vi "Variant Array to JSON Object text.vi"(5 "enable LabVIEW extensions? (T)":bool, 7 "Pretty Print?":bool, 8 "error in (no error)":errorcluster, 9 "Names":string[](array[string]), 10 "Array":variant[](array[variant])) -> (0 "error out":errorcluster, 3 "<JSON>Object Text":string)   [LabVIEW 2013, in "JSONtext.lvlib"]
uses:
  JSONtext.lvlib
  support/Tag for JSON Text.vi
  <vilib>/Utility/VariantDataType/VariantType.lvlib
  support/JSONtext support.lvlib
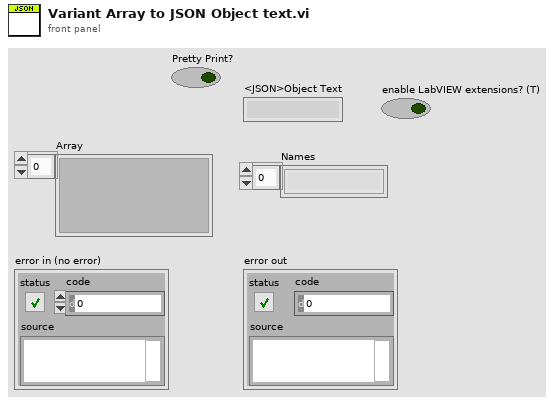
[diagram p1: front panel]
types:
  T1 = typedef "VariantType.lvlib/Type.ctl" = enum8{"Invalid Type", "Void", "I8", "I16", "I32", "I64", "U8", "U16", "U32", "U64", "Single Float", "Double Float", "Extended Float", "Single Complex", "Double Complex", "Extended Complex", "Enum U8", "Enum U16", "Enum U32", "Enum U64", "Single Float With Unit", "Double Float With Unit", "Extended Float With Unit", "Single Complex with Unit", "Double Complex with Unit", "Extended Complex with Unit", "Boolean", "String", "Path", "Picture", "Tag", "Array", "Cluster", "Variant", "LV Variant", "Waveform", "Timestamp", "Digital Waveform", "Digital Data", "ExpressData", "Refnum", "External Data", "VI", "Poly VI", "LabVIEW Class Instance", "Fixed Point"}
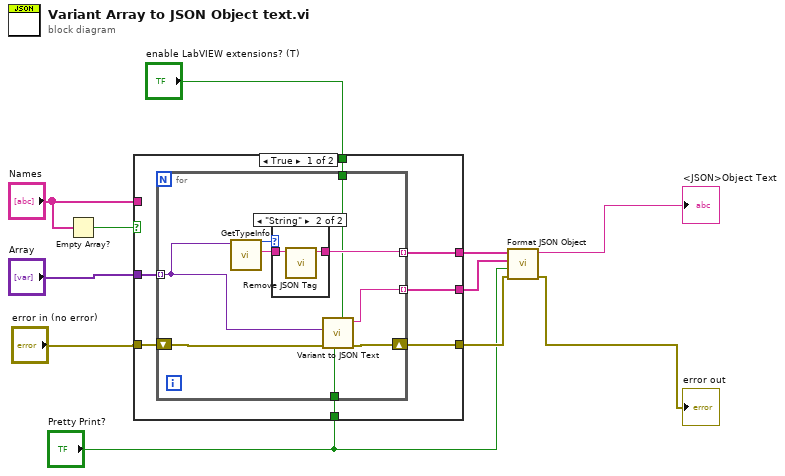
[diagram p0: block diagram]
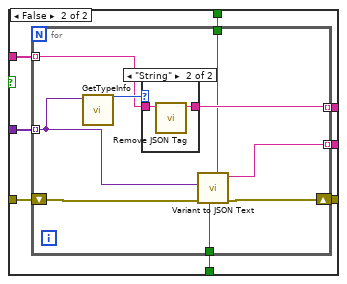
[diagram p3: hidden frame]
diagram:
  n1 = Empty Array?(array="Names") -> (empty?=w4:bool)
  n2 = case shown="True" w4 {
    tunnel: [w18 w38] -> w10
    tunnel: [w17 w37] -> w8
    tunnel: [w16 w36] -> w7
    tunnel: "error in (no error)" -> [w15 w35]
    tunnel: "Array" -> [w14 w34]
    tunnel: "Names" -> [_ w33]
    tunnel: "Pretty Print?" -> [w13 w32]
    tunnel: "enable LabVIEW extensions? (T)" -> [w12 w31]
    frame True {
      n3 = for {
        shift-right: [w23] -> w18
        shift-left: w15 -> [w24]
        tunnel: w14 -> [w27] mode=indexing
        tunnel: [w19] -> w17 mode=indexing
        tunnel: [w22] -> w16 mode=indexing
        tunnel: w13 -> [w21]
        tunnel: w12 -> [w20]
        n4 = call <vilib>:"GetTypeInfo.vi"("Variant"=w27) -> ("Name"=w25:string, "Type Enum"=w26:T1)  [unwired: 6 in, 3 out]
        n5 = case shown="\"String\"" w26 {
          tunnel: w25 -> [w28 w30]
          tunnel: [w28 w29] -> w22
          frame Default {
          }
          frame "String" {
            n6 = call "Remove JSON Tag.vi"("Name"=w30) -> ("Name (tag stripped)"=w29:string)  [unwired: 9 in, 1 out]
          }
        }
        n7 = call "Variant to JSON Text.vi"("enable LabVIEW extensions? (T)"=w20, "Pretty Print?"=w21, "error in (no error)"=w24, "Variant"=w27) -> ("error out"=w23:errorcluster, "<JSON>"=w19:string)  [unwired: 6 in]
      }
    }
    frame False {
      n8 = for {
        shift-right: [w44] -> w38
        shift-left: w35 -> [w45]
        tunnel: w34 -> [w47] mode=indexing
        tunnel: [w39] -> w37 mode=indexing
        tunnel: [w43] -> w36 mode=indexing
        tunnel: w33 -> [w42] mode=indexing
        tunnel: w32 -> [w41]
        tunnel: w31 -> [w40]
        n9 = call <vilib>:"GetTypeInfo.vi"("Variant"=w47) -> ("Type Enum"=w46:T1)  [unwired: 6 in, 4 out]
        n10 = case shown="\"String\"" w46 {
          tunnel: w42 -> [w48 w50]
          tunnel: [w48 w49] -> w43
          frame Default {
          }
          frame "String" {
            n11 = call "Remove JSON Tag.vi"("Name"=w50) -> ("Name (tag stripped)"=w49:string)  [unwired: 9 in, 1 out]
          }
        }
        n12 = call "Variant to JSON Text.vi"("enable LabVIEW extensions? (T)"=w40, "Pretty Print?"=w41, "error in (no error)"=w45, "Variant"=w47) -> ("error out"=w44:errorcluster, "<JSON>"=w39:string)  [unwired: 6 in]
      }
    }
  }
  n13 = call "Format JSON Object.vi"("error in (no error)"=w10, "Pretty Print?"="Pretty Print?", "JSON elements"=w8, "Names"=w7) -> ("error out"=→"error out":errorcluster, "JSON Object Text out"=→"<JSON>Object Text":string)  [unwired: 6 in]
